vi "校准日志.vi"(8 "error in (no error)":errorcluster, 10 "table":string="操作日志", 11 "日志信息":string) -> (0 "error out":errorcluster)   [LabVIEW 2016, in "斯坦道多参数.lvlib"]
uses:
  <vilib>/addons/database/Auxilliary.llb/DB Tools Transaction.ctl
  <vilib>/addons/database/Auxilliary.llb/DB Tools Isolation Level.ctl
  <vilib>/Utility/sysdir.llb/System Directory Type.ctl
  <vilib>/addons/database/Connection.llb/DB Tools Open Connec (String).vi
  <vilib>/addons/database/Connection.llb/Conn Transaction.vi
  <vilib>/addons/database/NI_Database_API.lvlib
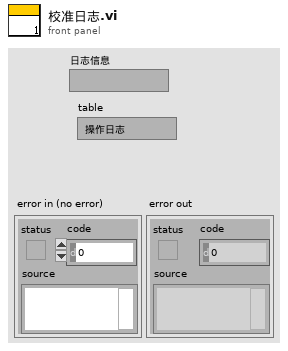
[diagram p1: front panel]
types:
  T1 = typedef "NI_Database_API.lvlib/DB Tools Isolation Level.ctl" = enum16{"chaos", "read uncommitted", "read committed", "repeatable read", "serializable"}
  T2 = typedef "NI_Database_API.lvlib/DB Tools Transaction.ctl" = enum16{"begin", "commit", "rollback"}
  T3 = cluster{"时间标识":timestamp, "设备":string, "日志信息":string, "流程参数":string}
  T4 = typedef "System Directory Type.ctl" = i32
  T5 = typedef "NI_Database_API.lvlib/Conn ObjectReference.ctl" = refnum<k1>
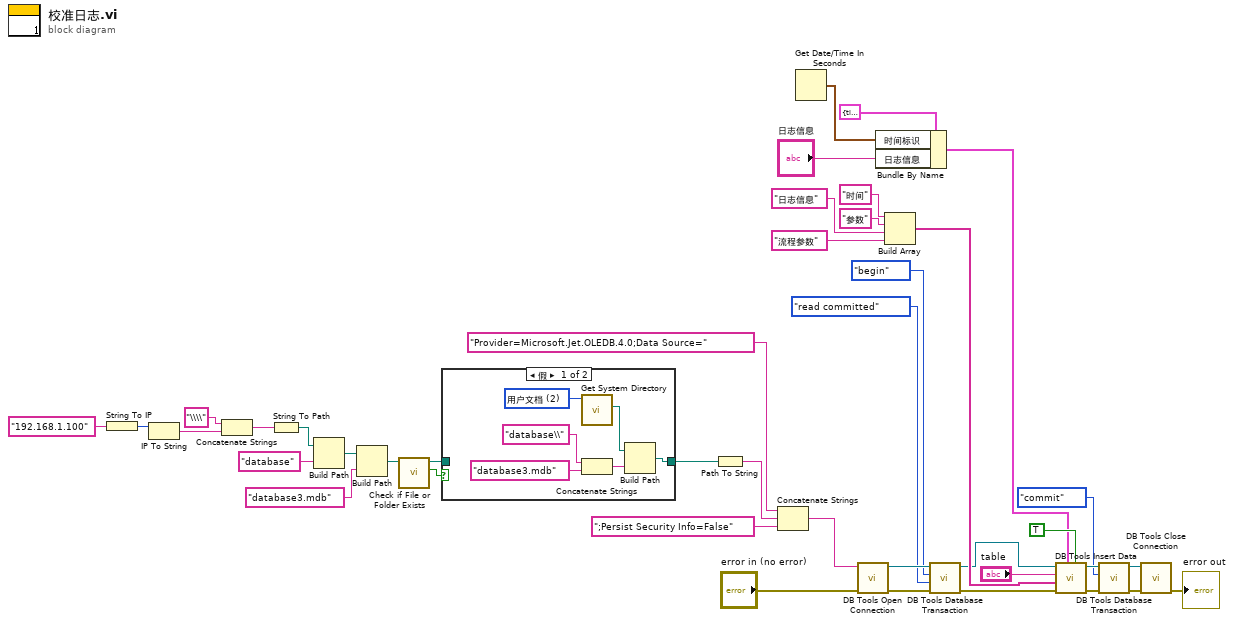
[diagram p0: block diagram]
diagram:
  n1 = String To IP(1:"192.168.1.100" ("名称")) -> (0:w15:u32)
  n2 = IP To String(2:w15) -> (0:w9:string)  [unwired: 1 in]
  n3 = Concatenate Strings("\\\\" ("字符串"), w9) -> (w12:string)
  n4 = String To Path(string=w12) -> (path=w14:path)
  n5 = Build Path(base path=w14, name or relative path="database" ("名称或相对路径")) -> (appended path=w10:path)
  n6 = Build Path(base path=w10, name or relative path="database3.mdb" ("database")) -> (appended path=w8:path)
  n7 = call <vilib>:"Check if File or Folder Exists.vi"("path"=w8) -> ("file or folder exists?"=w5:bool, "dup path"=w4:path)  [unwired: 8 in, 1 out]
  n8 = case shown="假" w5 {
    tunnel: w4 -> [_ w48]
    tunnel: [w42 w48] -> w3
    frame False {
      w43 = T4 2 items=["用户目录"=0, "用户桌面"=1, "用户文档"=2, "用户应用程序数据"=3, "用户设置"=4, "用户临时目录"=5, "公共文档"=6, "公共应用程序数据"=7, "公共设置"=8, "公共缓存"=13, "系统核心库"=9, "系统安装库"=10, "应用程序文件"=11, "启动盘根目录"=12] ("system directory type")
      n9 = call <vilib>:"Get System Directory.vi"("system directory type"=w43) -> ("system directory"=w44:path)  [unwired: 10 in]
      n10 = Concatenate Strings("database\\" ("condition"), "database3.mdb" ("database")) -> (w46:string)
      n11 = Build Path(base path=w44, name or relative path=w46) -> (appended path=w42:path)
    }
    frame True {
    }
  }
  n12 = Path To String(path=w3) -> (string=w35:string)
  n13 = Concatenate Strings("Provider=Microsoft.Jet.OLEDB.4.0;Data Source=" ("condition"), w35, ";Persist Security Info=False" ("condition")) -> (w33:string)
  n14 = Get Date/Time In Seconds() -> (seconds since 1Jan1904=w28:timestamp)
  n15 = call-poly <vilib>:"DB Tools Open Connection.vi"("error in (no error)"="error in (no error)", "connection information"=w33) -> ("error out"=w24:errorcluster, "connection reference"=w32:T5)  [unwired: 6 in]
  n16 = Bundle By Name(cluster=T3 {"时间标识"=timestamp(0 s since 1904-01-01), "设备"="多参数", "日志信息"="", "流程参数"=""} ("data in"), "时间标识"=w28, "日志信息"="日志信息") -> (w27:T3)
  n17 = Build Array("时间", "参数" ("元素"), "日志信息", "流程参数") -> (w30:string[])
  n18 = call-poly <vilib>:"DB Tools Database Transaction.vi"("error in (no error)"=w24, "isolation level (chaos)"=DB_Tools_Isolation_Level."read committed", "operation (begin)"=DB_Tools_Transaction."begin", "connection reference"=w32) -> ("error out"=w23:errorcluster, "connection reference out"=w25:T5)  [unwired: 2 in]
  n19 = call <vilib>:"DB Tools Insert Data.vi"("create table? (F)"=TRUE, "data"=w27, "error in (no error)"=w23, "columns"=w30, "table"="table", "connection reference"=w25) -> ("error out"=w20:errorcluster, "connection reference out"=w22:T5)  [unwired: 4 in]
  n20 = call-poly <vilib>:"DB Tools Database Transaction.vi"("error in (no error)"=w20, "operation (begin)"=DB_Tools_Transaction."commit", "connection reference"=w22) -> ("error out"=w19:errorcluster, "connection reference out"=w21:T5)  [unwired: 3 in]
  n21 = call <vilib>:"DB Tools Close Connection.vi"("error in (no error)"=w19, "connection reference"=w21) -> ("error out"=→"error out":errorcluster)  [unwired: 5 in]
